vi "Call and Forget.vi"(8 "Error In":errorcluster, 11 "Hook":path=path "") -> (0 "Error Out":errorcluster, 3 "Call and Forget":bool)   [LabVIEW 2018, in "Toolkit.lvlib"]
uses:
  Toolkit.lvlib
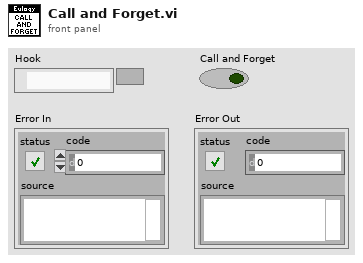
[diagram p1: front panel]
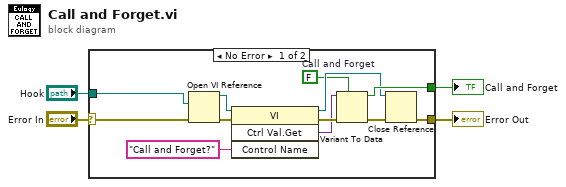
[diagram p0: block diagram]
diagram:
  n1 = case shown="No Error" "Error In" {
    selector: "Error In" -> [w5 w17]
    tunnel: "Hook" -> [w16 _]
    tunnel: [w15 _] -> w3
    tunnel: [w14 w17] -> w2
    frame No Error {
      w9 = FALSE  # Call and Forget
      n2 = Open VI Reference(vi path=w16, error in (no error)=w5) -> (vi reference=w11:refnum<vi>, error out=w10:errorcluster)  [unwired: 4 in]
      n3 = invoke class="VI" method="Ctrl Val.Get"(reference=w11, error in=w10, "Control Name"="Call and Forget?") -> (reference out=w13:refnum<vi>, error out=w8:errorcluster, "Get Control Value Variant"=w7:variant)  [unwired: 1 in, 1 out]
      n4 = Variant To Data(error in=w8, type=w9, Variant=w7) -> (data=w15:bool, error out=w12:errorcluster)
      n5 = Close Reference(reference=w13, error in (no error)=w12) -> (error out=w14:errorcluster)
    }
    frame Error {
    }
  }
  "Call and Forget" <- w3
  "Error Out" <- w2
